vi "Call_signal_fromHW.vi"(5 "Plot window":string) -> (0 "Y name":string, 1 "Y # signal":string, 2 "Ready?":bool)   [LabVIEW 2022 SP3]
doc: "Through this function you can select the stored signals from the Main_menu."
panel:
  out "Clone Name":string
  in  "Select signal":string(combo)
  in  "Add":bool
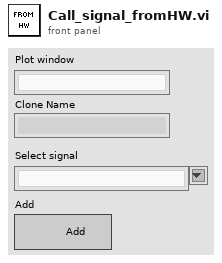
[diagram p1: front panel]
types:
  T1 = enum32{"Invalid", "Standard", "Closed", "Hidden", "Minimized", "Maximized"}
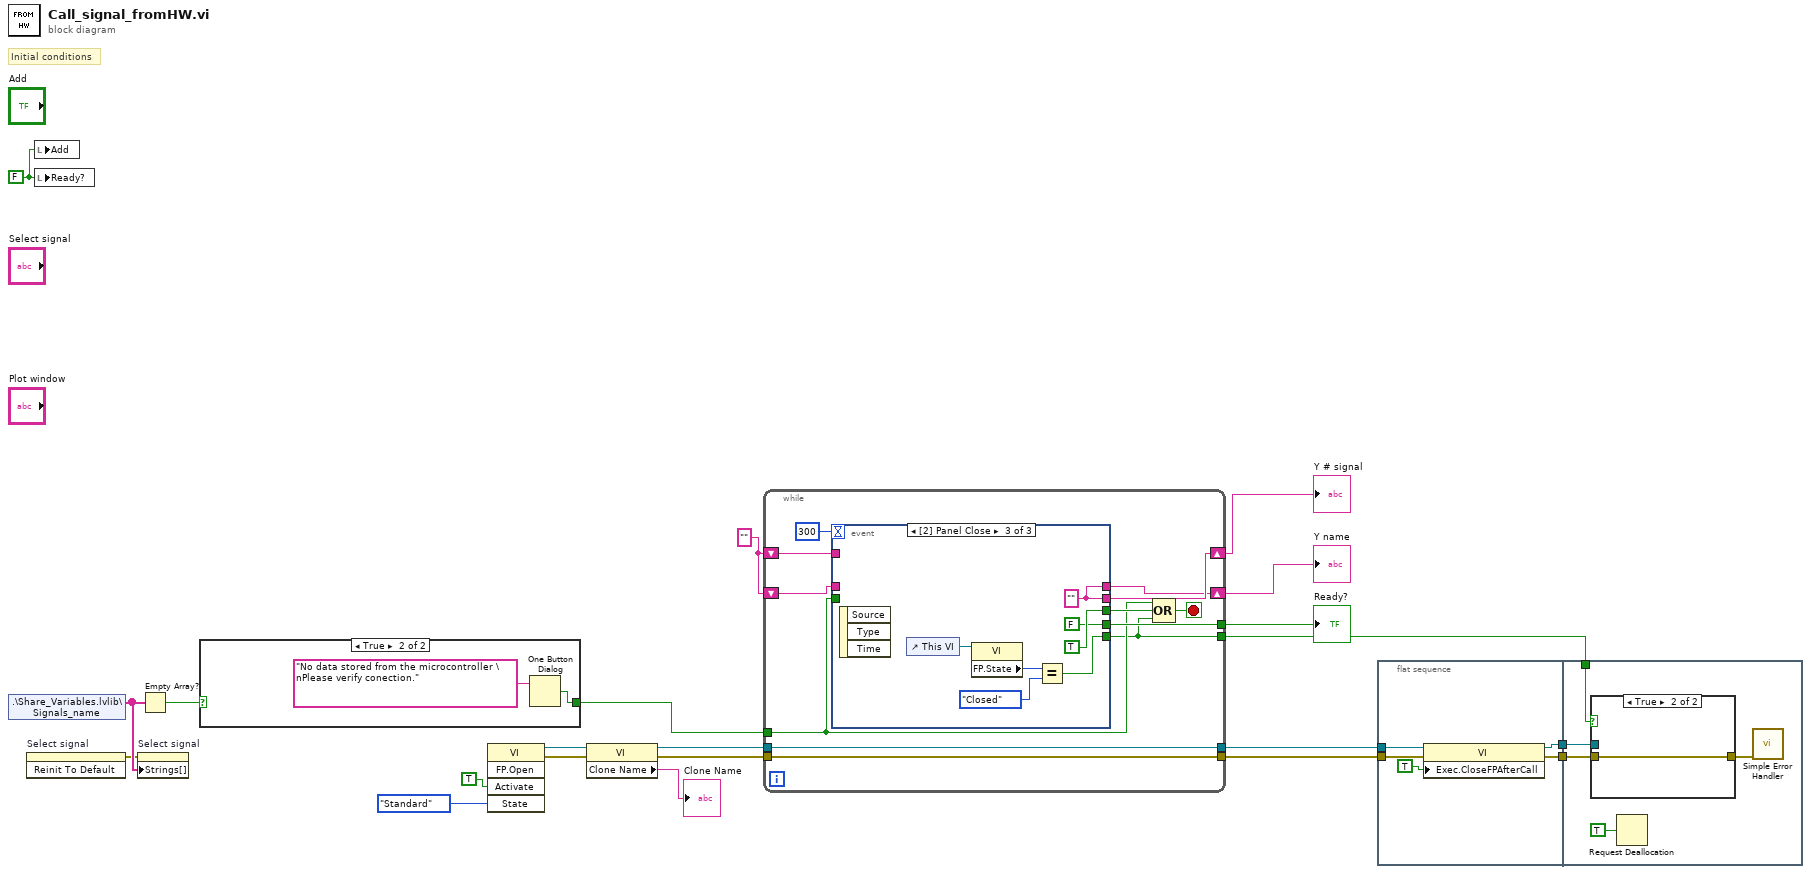
[diagram p0: block diagram]
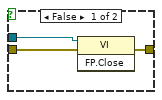
[diagram p3: hidden frame]
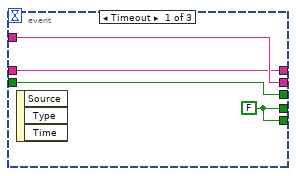
[diagram p4: hidden frame]
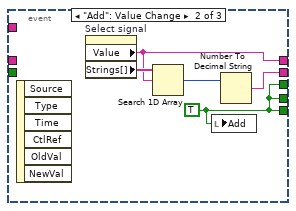
[diagram p5: hidden frame]
diagram:
  w4 = "" ("Value")
  w10 = FALSE
  # "Initial conditions"
  n1 = shared-variable ".\\Share_Variables.lvlib\\Signals_name"() -> (w9:string[])  [unwired: 1 in, 1 out]
  n2 = invoke on="Select signal" class="CmbBox" method="Reinit To Default"() -> (error out=w2:errorcluster)  [unwired: 3 in, 2 out]
  n3 = local write "Add"(w10) -> ()
  n4 = local write "Ready?"(w10) -> ()
  n5 = property on="Select signal" class="CmbBox"(error in=w2, "Strings[]"=w9) -> ()  [unwired: 1 in, 2 out]
  n6 = Empty Array?(array=w9) -> (empty?=w8:bool)
  n7 = case shown="True" w8 {
    selector: w8 -> [w22 _]
    tunnel: [w22 w23] -> w7
    frame False {
    }
    frame True {
      n8 = One Button Dialog(message="No data stored from the microcontroller \nPlease verify conection.") -> (true=w23:bool)  [unwired: 1 in]
    }
  }
  n9 = invoke on="Invoke Node" class="VI" method="FP.Open"("Activate"=TRUE ("Activate?"), "State"=T1."Standard") -> (reference out=w17:refnum<vi>, error out=w18:errorcluster)  [unwired: 3 in, 3 out]
  n10 = property on="Property Node" class="VI"(reference=w17, error in=w18) -> (reference out=w16:refnum<vi>, error out=w19:errorcluster, "Clone Name"=→"Clone Name":string)
  n11 = while {
    tunnel: [w36] -> w21
    tunnel: w19 -> [w35]
    tunnel: w16 -> [w30]
    tunnel: [w30] -> w14
    tunnel: [w35] -> w13
    tunnel: w7 -> [w28]
    shift-right: [w34] -> w5
    shift-left: w4 -> [w33]
    shift-right: [w32] -> w6
    shift-left: w4 -> [w31]
    tunnel: [w25] -> w1
    stop <- w27 stop-if-true
    n12 = event shown="[2] Panel Close" {
      selector: _ -> [_ _ _]
      dyn-events: _ -> [_ _ _]
      timeout: 300 -> [_ _ _]
      tunnel: [w38 w41 TRUE] -> w29
      tunnel: [w37 w41 FALSE] -> w36
      tunnel: [w40 w42 w47] -> w34
      tunnel: w33 -> [w40 _ _]
      tunnel: [w39 w43 w47] -> w32
      tunnel: w31 -> [w39 _ _]
      tunnel: w28 -> [w38 _ _]
      tunnel: [w37 w41 w46] -> w25
      event Timeout {
        w37 = FALSE
        n13 = event-data() -> ()  [unwired: 1 in, 3 out]
      }
      event "Add": Value Change {
        w41 = TRUE
        n14 = event-data() -> ()  [unwired: 1 in, 6 out]
        n15 = property on="Select signal" class="CmbBox"() -> ("Value"=w43:string, "Strings[]"=w45:string[])  [unwired: 2 in, 2 out]
        n16 = Search 1D Array(1D array=w45, element=w43) -> (index of element=w44:i32)  [unwired: 1 in]
        n17 = local write "Add"(w41) -> ()
        n18 = Number To Decimal String(number=w44) -> (decimal integer string=w42:string)  [unwired: 1 in]
      }
      event Panel Close {
        w47 = "" ("Value")
        n19 = event-data() -> ()  [unwired: 1 in, 3 out]
        n20 = control-ref of="This VI"() -> (w50:refnum<vi>)
        n21 = property class="VI"(reference=w50) -> ("FP.State"=w49:T1)  [unwired: 1 in, 2 out]
        n22 = Equal?(x=w49, y=T1."Closed" ("Front Panel Window:State")) -> (x = y?=w46:bool)
      }
    }
    n23 = Compound Arithmetic op=OR(w28, w29, w25) -> (w27:bool)
  }
  "Ready?" <- w21
  "Y name" <- w6
  "Y # signal" <- w5
  n24 = flat-sequence {
    tunnel: w14 -> [w57]
    tunnel: w13 -> [w56]
    tunnel: [w54] -> w12
    tunnel: [w53] -> w11
    tunnel: w12 -> [w61]
    tunnel: w11 -> [w60]
    tunnel: w1 -> [w58]
    frame #0 {
      n25 = property class="VI"(reference=w57, error in=w56, "Exec.CloseFPAfterCall"=TRUE ("Activate?")) -> (reference out=w54:refnum<vi>, error out=w53:errorcluster)
    }
    frame #1 {
      n26 = case shown="True" w58 {
        tunnel: [w65 w66] -> w62
        tunnel: w61 -> [w64 _]
        tunnel: w60 -> [w63 w66]
        frame False {
          n27 = invoke class="VI" method="FP.Close"(reference=w64, error in=w63) -> (error out=w65:errorcluster)  [unwired: 1 in, 2 out]
        }
        frame True {
        }
      }
      n28 = Request Deallocation(TRUE ("flag")) -> ()
      n29 = call <vilib>:"Simple Error Handler.vi"("error in (no error)"=w62) -> ()  [unwired: 4 in, 5 out]
    }
  }
